vi "Download Feed.vi"(8 "error in":errorcluster, 10 "destination folder":path, 11 "feed URI":string) -> (0 "error out":errorcluster)   [LabVIEW 2014, in "NIPM_API.lvlib"]
doc: "Downloads all packages from the specified feed URI to a destination folder.\n\nInputs:\nfeed URI - Specifies the feed URI of the feed.\nNote: If the feed URI is not currently registered, this VI will temporarily register the feed URI, download the packages in the feed, and then unregister the feed.\n\nDestination folder - Specifies the folder to place the downloaded package file(s) from the specified feed"
uses:
  NIPM_API.lvlib
panel:
  out "cmd standard output":string
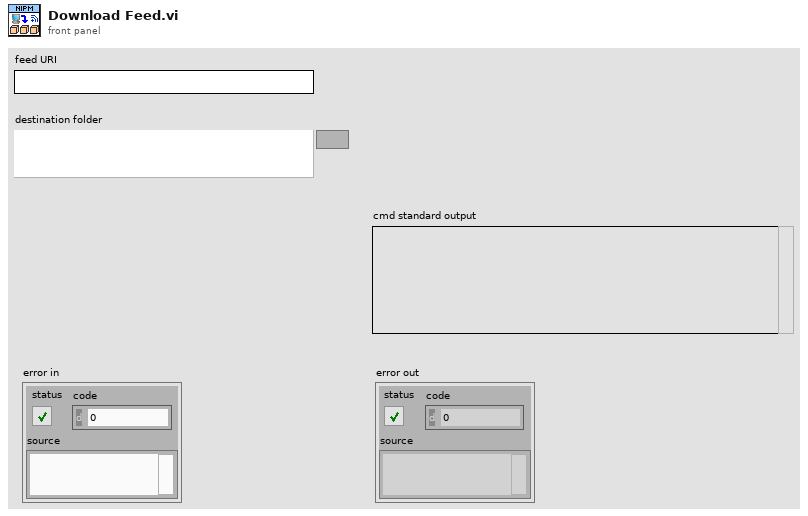
[diagram p1: front panel]
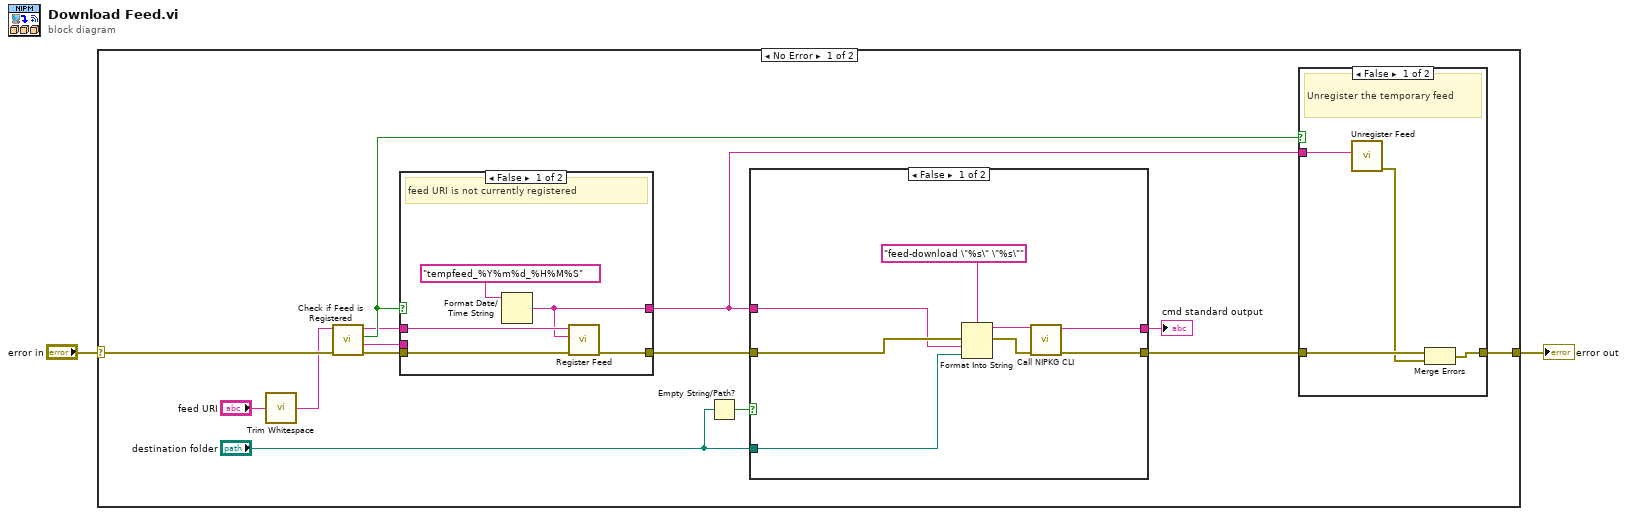
[diagram p0: block diagram]
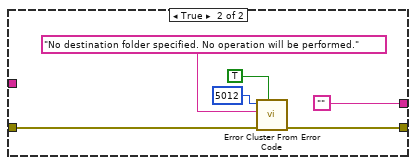
[diagram p2: hidden frame]
diagram:
  n1 = case shown="No Error" "error in" {
    selector: "error in" -> [w13 w43]
    tunnel: [w4 w43] -> w1
    frame No Error {
      n2 = call <vilib>:"Trim Whitespace.vi"("string"="feed URI") -> ("trimmed string"=w12:string)  [unwired: 1 in]
      n3 = call "Check if Feed is Registered.vi"("error in"=w13, "feed URI"=w12) -> ("error out"=w11:errorcluster, "feed name"=w7:string, "feed URI registered?"=w9:bool, "feed URI out"=w8:string)  [unwired: 6 in]
      n4 = case shown="False" w9 {
        tunnel: w11 -> [w40 w42]
        tunnel: [w39 w42] -> w10
        tunnel: w8 -> [w38 _]
        tunnel: [w36 w41] -> w5
        tunnel: w7 -> [_ w41]
        frame False {
          # "feed URI is not currently registered"
          n5 = Format Date/Time String(time format string (%c)="tempfeed_%Y%m%d_%H%M%S") -> (date/time string=w36:string)  [unwired: 2 in]
          n6 = call "Register Feed.vi"("error in"=w40, "feed name"=w36, "feed URI"=w38) -> ("error out"=w39:errorcluster)  [unwired: 7 in, 1 out]
        }
        frame True {
          # "feed URI is already registered"
        }
      }
      n7 = Empty String/Path?(string/path="destination folder") -> (empty?=w6:bool)
      n8 = case shown="False" w6 {
        tunnel: w10 -> [w24 w27]
        tunnel: [w21 w26] -> w3
        tunnel: [w20 ""] -> w14
        tunnel: "destination folder" -> [w19 _]
        tunnel: w5 -> [w17 _]
        frame False {
          n9 = Format Into String(format string="feed-download \"%s\" \"%s\"", error in=w24, w17, w19) -> (resulting string=w23:string, error out=w22:errorcluster)  [unwired: 1 in]
          n10 = call "Call NIPKG CLI.vi"("error in (no error)"=w22, "command"=w23) -> ("error out"=w21:errorcluster, "command line standard output"=w20:string)  [unwired: 8 in]
        }
        frame True {
          n11 = call <vilib>:"Error Cluster From Error Code.vi"("show call chain? (False)"=TRUE, "error in (no error)"=w27, "error message (\"\")"="No destination folder specified. No operation will be performed.", "error code (0)"=5012) -> ("error out"=w26:errorcluster)  [unwired: 5 in]
        }
      }
      "cmd standard output" <- w14
      n12 = case shown="False" w9 {
        tunnel: w5 -> [w34 _]
        tunnel: [w32 w35] -> w4
        tunnel: w3 -> [w33 w35]
        frame False {
          # "Unregister the temporary feed"
          n13 = call "Unregister Feed.vi"("feed name"=w34) -> ("error out"=w31:errorcluster)  [unwired: 9 in, 1 out]
          n14 = Merge Errors(w33, w31) -> (w32:errorcluster)
        }
        frame True {
          # "Do nothing.  No temporary feeds were registered."
        }
      }
    }
    frame Error {
    }
  }
  "error out" <- w1
